vi "tunable_lenses.vi"(8 "DAC4":u16, 9 "DAC3":u16, 10 "DAC2":u16, 11 "DAC1":u16) -> (2 "Digital Waveform Graph":digitalwaveform[](graph))   [LabVIEW 2013]
uses:
  <vilib>/Utility/error.llb/DialogType.ctl
  <vilib>/DAQmx/write.llb/DAQmx Write (Digital 1D Wfm NChan NSamp).vi
  <vilib>/Waveform/DWDTOps.llb/Digital Pattern Generator (Single Value).vi
  <vilib>/Waveform/DWDTOps.llb/DWDT Append Digital Samples.vi
  <vilib>/Waveform/DWDTOps.llb/DWDT Digital Size.vi
  <vilib>/DAQmx/create/channels.llb/DAQmx Create Channel (DO-Digital Output).vi
  <vilib>/DAQmx/configure/timing.llb/DAQmx Timing (Sample Clock).vi
  <vilib>/Waveform/DWDTOps.llb/DWDT Uncompress Digital.vi
  <vilib>/DAQmx/miscellaneous.llb/DAQmx Fill In Error Info.vi
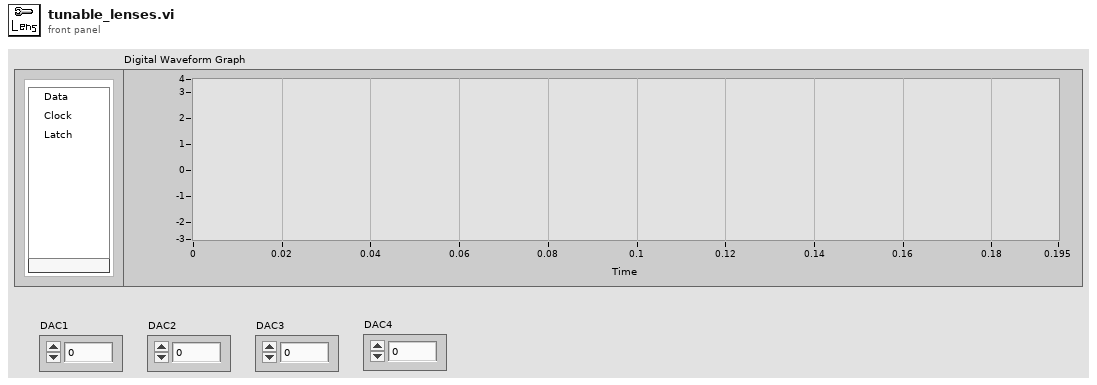
[diagram p1: front panel]
types:
  T1 = typedef "DialogType.ctl" = u16
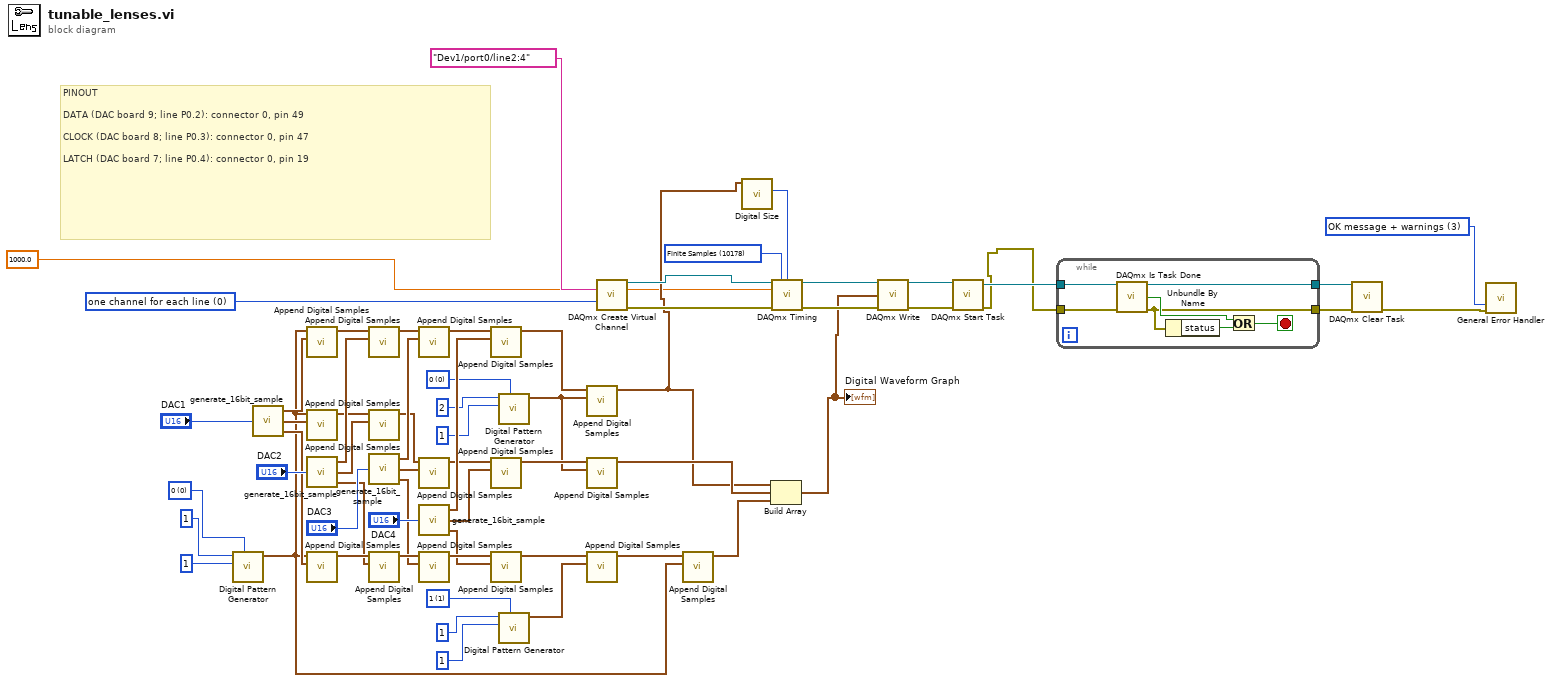
[diagram p0: block diagram]
diagram:
  w4 = 10178 items=["Finite Samples"=10178, "Continuous Samples"=10123, "Hardware Timed Single Point"=12522] ("sample mode")
  w10 = 0 items=["one channel for each line", "one channel for all lines"] ("line grouping")
  w16 = u8 1 items=["0", "1", "Z", "L", "H", "X", "T", "V"] ("value")
  w24 = u8 0 items=["0", "1", "Z", "L", "H", "X", "T", "V"] ("value")
  w48 = u8 0 items=["0", "1", "Z", "L", "H", "X", "T", "V"] ("value")
  w53 = T1 3 items=["no dialog", "OK message", "continue or stop message", "OK message + warnings", "continue/stop + warnings"] ("type of dialog (OK msg:1)")
  # "PINOUT\n\nDATA (DAC board 9; line P0.2): connector 0, pin 49\n\nCLOCK (DAC board 8; line P0.3): connector 0, pin 47\n\nLATCH (DAC board 7; line P0.4): connector 0, pin 19"
  n1 = call-poly <vilib>:"Digital Pattern Generator.vi"("value"=w48, "number of signals"=u32 1, "number of samples"=u32 1) -> ("digital waveform"=w12:digitalwaveform)  [unwired: 7 in, 1 out]
  n2 = call "generate_16bit_sample.vi"("Value"="DAC1") -> ("latch"=w28:digitalwaveform, "clock"=w38:digitalwaveform, "data"=w45:digitalwaveform)  [unwired: 2 in]
  n3 = call-poly <vilib>:"Append Digital Samples.vi"("digital waveform B"=w45, "digital waveform A"=w12) -> ("digital waveform out"=w44:digitalwaveform)  [unwired: 8 in, 1 out]
  n4 = call-poly <vilib>:"Append Digital Samples.vi"("digital waveform B"=w38, "digital waveform A"=w12) -> ("digital waveform out"=w37:digitalwaveform)  [unwired: 8 in, 1 out]
  n5 = call "generate_16bit_sample.vi"("Value"="DAC2") -> ("latch"=w27:digitalwaveform, "clock"=w36:digitalwaveform, "data"=w43:digitalwaveform)  [unwired: 2 in]
  n6 = call-poly <vilib>:"Append Digital Samples.vi"("digital waveform B"=w28, "digital waveform A"=w12) -> ("digital waveform out"=w31:digitalwaveform)  [unwired: 8 in, 1 out]
  n7 = call-poly <vilib>:"Append Digital Samples.vi"("digital waveform B"=w43, "digital waveform A"=w44) -> ("digital waveform out"=w41:digitalwaveform)  [unwired: 8 in, 1 out]
  n8 = call-poly <vilib>:"Append Digital Samples.vi"("digital waveform B"=w36, "digital waveform A"=w37) -> ("digital waveform out"=w35:digitalwaveform)  [unwired: 8 in, 1 out]
  n9 = call "generate_16bit_sample.vi"("Value"="DAC3") -> ("latch"=w26:digitalwaveform, "clock"=w34:digitalwaveform, "data"=w42:digitalwaveform)  [unwired: 2 in]
  n10 = call-poly <vilib>:"Append Digital Samples.vi"("digital waveform B"=w27, "digital waveform A"=w31) -> ("digital waveform out"=w30:digitalwaveform)  [unwired: 8 in, 1 out]
  n11 = call-poly <vilib>:"Append Digital Samples.vi"("digital waveform B"=w42, "digital waveform A"=w41) -> ("digital waveform out"=w39:digitalwaveform)  [unwired: 8 in, 1 out]
  n12 = call-poly <vilib>:"Append Digital Samples.vi"("digital waveform B"=w34, "digital waveform A"=w35) -> ("digital waveform out"=w32:digitalwaveform)  [unwired: 8 in, 1 out]
  n13 = call "generate_16bit_sample.vi"("Value"="DAC4") -> ("latch"=w25:digitalwaveform, "clock"=w33:digitalwaveform, "data"=w40:digitalwaveform)  [unwired: 2 in]
  n14 = call-poly <vilib>:"Append Digital Samples.vi"("digital waveform B"=w26, "digital waveform A"=w30) -> ("digital waveform out"=w29:digitalwaveform)  [unwired: 8 in, 1 out]
  n15 = call-poly <vilib>:"Append Digital Samples.vi"("digital waveform B"=w40, "digital waveform A"=w39) -> ("digital waveform out"=w21:digitalwaveform)  [unwired: 8 in, 1 out]
  n16 = call-poly <vilib>:"Append Digital Samples.vi"("digital waveform B"=w33, "digital waveform A"=w32) -> ("digital waveform out"=w20:digitalwaveform)  [unwired: 8 in, 1 out]
  n17 = call-poly <vilib>:"Append Digital Samples.vi"("digital waveform B"=w25, "digital waveform A"=w29) -> ("digital waveform out"=w18:digitalwaveform)  [unwired: 8 in, 1 out]
  n18 = call-poly <vilib>:"Digital Pattern Generator.vi"("value"=w24, "number of signals"=u32 1, "number of samples"=u32 2) -> ("digital waveform"=w19:digitalwaveform)  [unwired: 7 in, 1 out]
  n19 = call-poly <vilib>:"Digital Pattern Generator.vi"("value"=w16, "number of signals"=u32 1, "number of samples"=u32 1) -> ("digital waveform"=w13:digitalwaveform)  [unwired: 7 in, 1 out]
  n20 = call-poly <vilib>:"Append Digital Samples.vi"("digital waveform B"=w19, "digital waveform A"=w21) -> ("digital waveform out"=w8:digitalwaveform)  [unwired: 8 in, 1 out]
  n21 = call-poly <vilib>:"Append Digital Samples.vi"("digital waveform B"=w19, "digital waveform A"=w20) -> ("digital waveform out"=w9:digitalwaveform)  [unwired: 8 in, 1 out]
  n22 = call-poly <vilib>:"Append Digital Samples.vi"("digital waveform B"=w13, "digital waveform A"=w18) -> ("digital waveform out"=w17:digitalwaveform)  [unwired: 8 in, 1 out]
  n23 = call-poly <vilib>:"DAQmx Create Virtual Channel.vi"("lines"=tag "Dev1/port0/line2:4", "line grouping"=w10) -> ("task out"=w61:refnum<k21>, "error out"=w60:errorcluster)  [unwired: 5 in, 7 out]
  n24 = call-poly <vilib>:"Append Digital Samples.vi"("digital waveform B"=w12, "digital waveform A"=w17) -> ("digital waveform out"=w11:digitalwaveform)  [unwired: 8 in, 1 out]
  n25 = call-poly <vilib>:"Digital Size.vi"("digital waveform in"=w8) -> ("number of samples"=w7:i32)  [unwired: 7 in, 3 out]
  n26 = Build Array(w8, w9, w11) -> (w3:digitalwaveform[])
  "Digital Waveform Graph" <- w3
  n27 = call-poly <vilib>:"DAQmx Timing.vi"("task/channels in"=w61, "sample mode"=w4, "samples per channel"=w7, "rate"=1000.0, "error in"=w60) -> ("task out"=w6:refnum<k21>, "error out"=w59:errorcluster)  [unwired: 2 in, 7 out]
  n28 = call-poly <vilib>:"DAQmx Write.vi"("task/channels in"=w6, "data"=w3, "error in"=w59) -> ("task out"=w58:refnum<k21>, "error out"=w57:errorcluster)  [unwired: 2 in, 9 out]
  n29 = call <vilib>:"DAQmx Start Task.vi"("task/channels in"=w58, "error in"=w57) -> ("task out"=w56:refnum<k21>, "error out"=w2:errorcluster)  [unwired: 12 out]
  n30 = while {
    tunnel: w56 -> [w69]
    tunnel: w2 -> [w68]
    tunnel: [w64] -> w55
    tunnel: [w63] -> w54
    stop <- w65 stop-if-true
    n31 = call <vilib>:"DAQmx Is Task Done.vi"("task/channels in"=w69, "error in"=w68) -> ("task out"=w64:refnum<k21>, "task done?"=w66:bool, "error out"=w63:errorcluster)  [unwired: 2 in, 9 out]
    n32 = Unbundle By Name(w63) -> ("status"=w67:bool)
    n33 = Or(x=w66, y=w67) -> (x .or. y?=w65:bool)
  }
  n34 = call <vilib>:"DAQmx Clear Task.vi"("task in"=w55, "error in"=w54) -> ("error out"=w1:errorcluster)  [unwired: 13 out]
  n35 = call <vilib>:"General Error Handler.vi"("type of dialog (OK msg:1)"=w53, "error in (no error)"=w1) -> ()  [unwired: 14 out]
